vi "Serialize.vi"(8 "error in (no error)":errorcluster, 10 "Element in":refnum<k20>, 11 "Test Suite in":refnum<class "Test Suite.lvclass">) -> (0 "error out":errorcluster, 2 "Element out":refnum<k20>)   [LabVIEW 2013, in "JUnit XML.lvlib" / "Test Suite.lvclass"]
uses:
  Test Suite.lvclass
  Test Case/Test Result.ctl
  Test Suite.lvclass/Test Suite.ctl
  <vilib>/xml/Close Reference(Node).vi
  XML/XML.lvlib
  JUnit XML.lvlib
  <vilib>/xml/NI_XML.lvlib
  Test Case/Test Case.lvclass
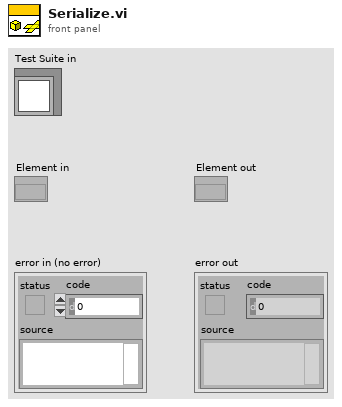
[diagram p1: front panel]
types:
  T1 = typedef "JUnit XML.lvlib/Test Case.lvclass/Test Result.ctl" = enum16{"Success", "Failure", "Error", "Skipped"}
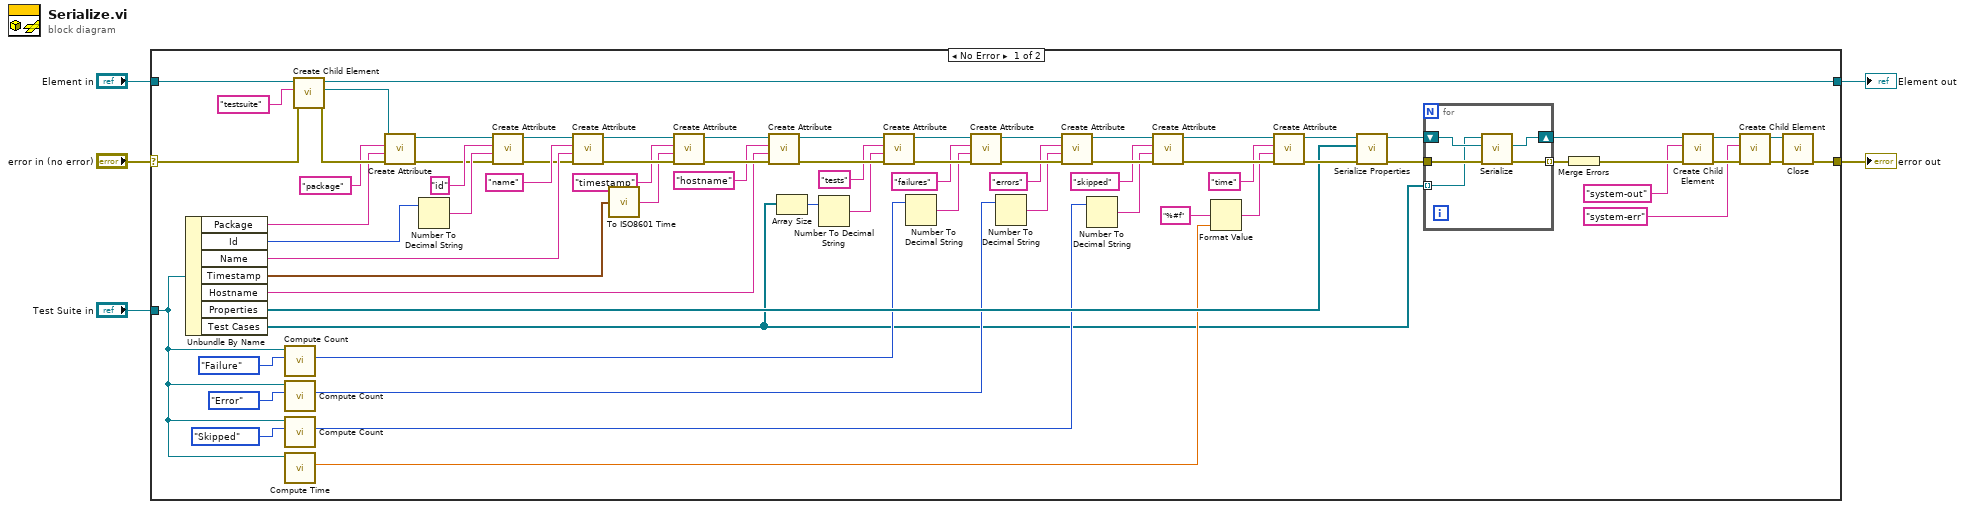
[diagram p0: block diagram]
diagram:
  n1 = case shown="No Error" "error in (no error)" {
    selector: "error in (no error)" -> [w33 w84]
    tunnel: [w18 w84] -> w4
    tunnel: "Test Suite in" -> [w10 _]
    tunnel: "Element in" -> [w32 w83]
    tunnel: [w31 w83] -> w1
    frame No Error {
      n2 = Unbundle By Name(w10) -> ("Package"=w34:string, "Id"=w41:i32, "Name"=w75:string, "Timestamp"=w71:timestamp, "Hostname"=w40:string, "Properties"=w17:refnum<class "Property.lvclass">[], "Test Cases"=w6:refnum<class "Test Case.lvclass">[])
      n3 = call "Compute Count.vi"("Test Result"=Test_Result."Failure", "Test Suite in"=w10) -> ("Count"=w8:i32)  [unwired: 7 in, 2 out]
      n4 = call "Compute Count.vi"("Test Result"=Test_Result."Error", "Test Suite in"=w10) -> ("Count"=w9:i32)  [unwired: 7 in, 2 out]
      n5 = call "Compute Count.vi"("Test Result"=Test_Result."Skipped", "Test Suite in"=w10) -> ("Count"=w14:i32)  [unwired: 7 in, 2 out]
      n6 = call "Compute Time.vi"("Test Suite in"=w10) -> ("Time"=w15:dbl)  [unwired: 8 in, 2 out]
      n7 = call "Create Child Element.vi"("error in (no error)"=w33, "Name"="testsuite" ("Tag Name"), "Element in"=w32) -> ("error out"=w38:errorcluster, "Child Element"=w37:refnum<k20>, "Element out"=w31:refnum<k20>)  [unwired: 6 in]
      n8 = call "Create Attribute.vi"("error in (no error)"=w38, "Value"=w34, "Name"="package" ("Attribute Name"), "Element in"=w37) -> ("error out"=w39:errorcluster, "Element out"=w36:refnum<k20>)  [unwired: 6 in]
      n9 = Number To Decimal String(number=w41) -> (decimal integer string=w42:string)  [unwired: 1 in]
      n10 = call "Create Attribute.vi"("error in (no error)"=w39, "Value"=w42, "Name"="id" ("Attribute Name"), "Element in"=w36) -> ("error out"=w45:errorcluster, "Element out"=w44:refnum<k20>)  [unwired: 6 in]
      n11 = call "Create Attribute.vi"("error in (no error)"=w45, "Value"=w75, "Name"="name" ("Attribute Name"), "Element in"=w44) -> ("error out"=w73:errorcluster, "Element out"=w74:refnum<k20>)  [unwired: 6 in]
      n12 = call "To ISO8601 Time.vi"("Time Stamp"=w71) -> ("String"=w70:string)  [unwired: 1 in]
      n13 = call "Create Attribute.vi"("error in (no error)"=w73, "Value"=w70, "Name"="timestamp" ("Attribute Name"), "Element in"=w74) -> ("error out"=w68:errorcluster, "Element out"=w69:refnum<k20>)  [unwired: 6 in]
      n14 = call "Create Attribute.vi"("error in (no error)"=w68, "Value"=w40, "Name"="hostname" ("Attribute Name"), "Element in"=w69) -> ("error out"=w65:errorcluster, "Element out"=w66:refnum<k20>)  [unwired: 6 in]
      n15 = Array Size(array=w6) -> (size(s)=w7:i32)
      n16 = Number To Decimal String(number=w7) -> (decimal integer string=w63:string)  [unwired: 1 in]
      n17 = call "Create Attribute.vi"("error in (no error)"=w65, "Value"=w63, "Name"="tests" ("Attribute Name"), "Element in"=w66) -> ("error out"=w62:errorcluster, "Element out"=w61:refnum<k20>)  [unwired: 6 in]
      n18 = Number To Decimal String(number=w8) -> (decimal integer string=w59:string)  [unwired: 1 in]
      n19 = call "Create Attribute.vi"("error in (no error)"=w62, "Value"=w59, "Name"="failures" ("Attribute Name"), "Element in"=w61) -> ("error out"=w57:errorcluster, "Element out"=w58:refnum<k20>)  [unwired: 6 in]
      n20 = Number To Decimal String(number=w9) -> (decimal integer string=w55:string)  [unwired: 1 in]
      n21 = call "Create Attribute.vi"("error in (no error)"=w57, "Value"=w55, "Name"="errors" ("Attribute Name"), "Element in"=w58) -> ("error out"=w53:errorcluster, "Element out"=w54:refnum<k20>)  [unwired: 6 in]
      n22 = Number To Decimal String(number=w14) -> (decimal integer string=w51:string)  [unwired: 1 in]
      n23 = call "Create Attribute.vi"("error in (no error)"=w53, "Value"=w51, "Name"="skipped" ("Attribute Name"), "Element in"=w54) -> ("error out"=w49:errorcluster, "Element out"=w50:refnum<k20>)  [unwired: 6 in]
      n24 = Format Value(format string="%#f", value (0)=w15) -> (output string=w46:string)  [unwired: 1 in]
      n25 = call "Create Attribute.vi"("error in (no error)"=w49, "Value"=w46, "Name"="time" ("Attribute Name"), "Element in"=w50) -> ("error out"=w19:errorcluster, "Element out"=w16:refnum<k20>)  [unwired: 6 in]
      n26 = call "Serialize Properties.vi"("error in (no error)"=w19, "Properties"=w17, "Node in"=w16) -> ("error out"=w28:errorcluster, "Node out"=w29:refnum<k20>)  [unwired: 7 in]
      n27 = for {
        tunnel: [w80] -> w30 mode=indexing
        tunnel: w28 -> [w79]
        shift-right: [w81] -> w27
        shift-left: w29 -> [w82]
        tunnel: w6 -> [w78] mode=indexing
        n28 = call "Serialize.vi"("error in (no error)"=w79, "Element in"=w82, "Test Case in"=w78) -> ("error out"=w80:errorcluster, "Element out"=w81:refnum<k20>)  [unwired: 7 in]
      }
      n29 = Merge Errors(w30) -> (w26:errorcluster)
      n30 = call "Create Child Element.vi"("error in (no error)"=w26, "Name"="system-out" ("Tag Name"), "Element in"=w27) -> ("error out"=w24:errorcluster, "Element out"=w25:refnum<k20>)  [unwired: 6 in, 1 out]
      n31 = call "Create Child Element.vi"("error in (no error)"=w24, "Name"="system-err" ("Tag Name"), "Element in"=w25) -> ("error out"=w23:errorcluster, "Element out"=w22:refnum<k20>)  [unwired: 6 in, 1 out]
      n32 = call-poly <vilib>:"Close.vi"("error in (no error)"=w23, "node"=w22) -> ("error out"=w18:errorcluster)  [unwired: 7 in]
    }
    frame Error {
    }
  }
  "error out" <- w4
  "Element out" <- w1
